vi "Overload.vi"(8 "INPUT2 Range":dbl, 9 "INPUT1 Range":dbl, 10 "CH1":dbl[](array[numeric]), 11 "INPUT 1":dbl[](array[numeric])) -> (0 "CH1 MIN":dbl, 1 "CH0 MIN":dbl, 2 "CH0 MAX":dbl, 3 "OL INPUT1":bool, 4 "CH1 MAX":dbl, 6 "OL CH1":bool)   [LabVIEW 2012]
panel:
  out "CH1 MIN INDEX":dbl
  out "CH1 MAX INDEX":dbl
  out "CH0 MIN INDEX":dbl
  out "CH0 MAX INDEX":dbl
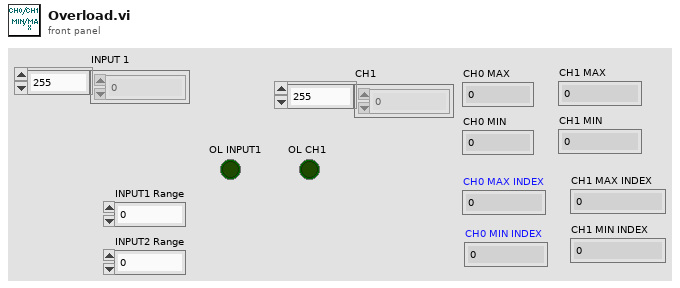
[diagram p1: front panel]
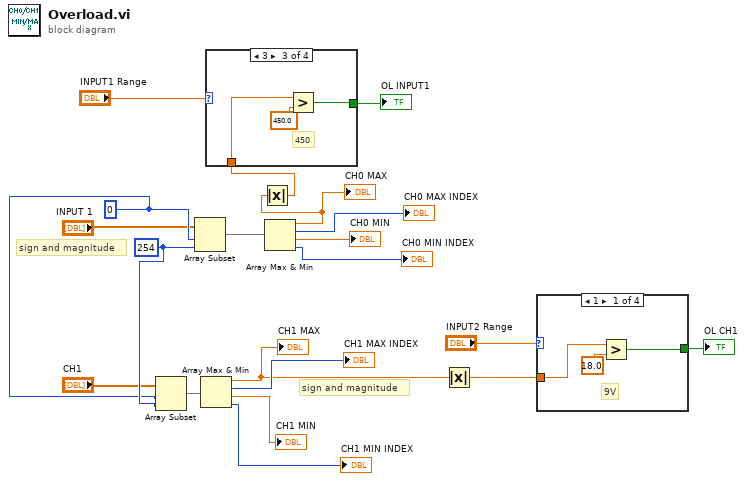
[diagram p0: block diagram]
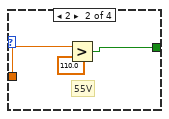
[diagram p2: hidden frame]
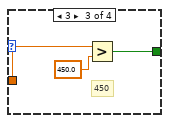
[diagram p3: hidden frame]
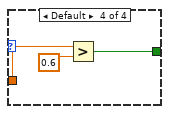
[diagram p4: hidden frame]
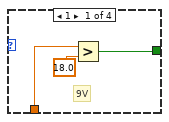
[diagram p5: hidden frame]
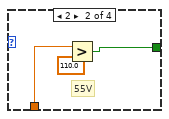
[diagram p6: hidden frame]
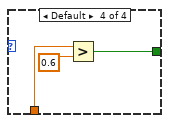
[diagram p7: hidden frame]
diagram:
  w11 = 0
  w12 = 254
  # "sign and magnitude"
  # "sign and magnitude"
  n1 = Array Subset(array="CH1", index=w11, length=w12) -> (w13:dbl[])
  n2 = Array Subset(array="INPUT 1", index=w11, length=w12) -> (w14:dbl[])
  n3 = Array Max & Min(array=w13) -> (max value=w3:dbl, max index (indices)=→"CH1 MAX INDEX":i32, min value=→"CH1 MIN":dbl, min index (indices)=→"CH1 MIN INDEX":i32)
  "CH1 MAX" <- w3
  n4 = Array Max & Min(array=w14) -> (max value=w4:dbl, max index (indices)=→"CH0 MAX INDEX":i32, min value=→"CH0 MIN":dbl, min index (indices)=→"CH0 MIN INDEX":i32)
  "CH0 MAX" <- w4
  n5 = Absolute Value(x=w4) -> (abs(x)=w5:dbl)
  n6 = case shown="3" "INPUT1 Range" {
    tunnel: w5 -> [w22 w26 w27 w32]
    tunnel: [w23 w24 w28 w30] -> w10
    frame 1 {
      # "9V"
      n7 = Greater?(x=w22, y=18.0) -> (0:w23:bool)
    }
    frame 2 {
      # "55V"
      n8 = Greater?(x=w26, y=110.0) -> (0:w24:bool)
    }
    frame 3 {
      # "450"
      n9 = Greater?(x=w27, y=450.0) -> (0:w28:bool)
    }
    frame Default {
      n10 = Greater?(x=w32, y=0.6) -> (0:w30:bool)
    }
  }
  "OL INPUT1" <- w10
  n11 = Absolute Value(x=w3) -> (abs(x)=w2:dbl)
  n12 = case shown="1" "INPUT2 Range" {
    tunnel: w2 -> [w33 w38 w39 w44]
    tunnel: [w35 w36 w40 w42] -> w6
    frame 1 {
      # "9V"
      n13 = Greater?(x=w33, y=18.0) -> (0:w35:bool)
    }
    frame 2 {
      # "55V"
      n14 = Greater?(x=w38, y=110.0) -> (0:w36:bool)
    }
    frame 3 {
      # "450"
      n15 = Greater?(x=w39, y=450.0) -> (0:w40:bool)
    }
    frame Default {
      n16 = Greater?(x=w44, y=0.6) -> (0:w42:bool)
    }
  }
  "OL CH1" <- w6
